vi "PPSU Feedback.vi"(8 "Error in":errorcluster, 11 "All Queue":T1) -> ()   [LabVIEW 2022 SP3]
uses:
  Controls/All Queue Ref.ctl
  Controls/PPSU Feedback ctl.ctl
  Controls/ALL Health.ctl
  6D_Global.vi
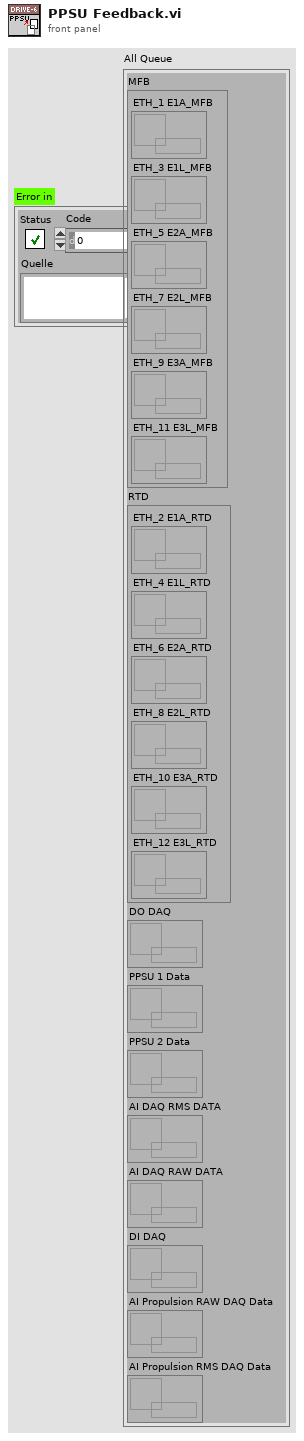
[diagram p1: front panel]
types:
  T1 = typedef "All Queue Ref.ctl" = cluster{"MFB":cluster{"ETH_1 E1A_MFB":refnum<queue>, "ETH_3 E1L_MFB":refnum<queue>, "ETH_5 E2A_MFB":refnum<queue>, "ETH_7 E2L_MFB":refnum<queue>, "ETH_9 E3A_MFB":refnum<queue>, "ETH_11 E3L_MFB":refnum<queue>}, "RTD":cluster{"ETH_2 E1A_RTD ":refnum<queue>, "ETH_4 E1L_RTD ":refnum<queue>, "ETH_6 E2A_RTD ":refnum<queue>, "ETH_8 E2L_RTD ":refnum<queue>, "ETH_10 E3A_RTD ":refnum<queue>, "ETH_12 E3L_RTD ":refnum<queue>}, "DO DAQ":refnum<queue>, "PPSU 1 Data":refnum<queue>, "PPSU 2 Data":refnum<queue>, "AI DAQ RMS DATA":refnum<queue>, "AI DAQ RAW DATA":refnum<queue>, "DI DAQ":refnum<queue>, "AI Propulsion RAW DAQ Data":refnum<queue>, "AI Propulsion RMS DAQ Data":refnum<queue>}
  T2 = typedef "PPSU Feedback ctl.ctl" = enum16{"Initialize", "Poll", "Read", "Exit"}
  T3 = typedef "ALL Health.ctl" = enum16{"AI HS", "AI 20kHZ HS", "DO HS", "Datalog HS", "PPSU HS", "ETH_1 DAQ", "ETH_1 RTD", "ETH_2 DAQ", "ETH_2 RTD", "ETH_5 RTD"}
  T4 = enum16{"Init", "Read 'All'", "Read 'n'", "Read '1'", "Write '1'", "Write 'n'", "Write 'All'"}
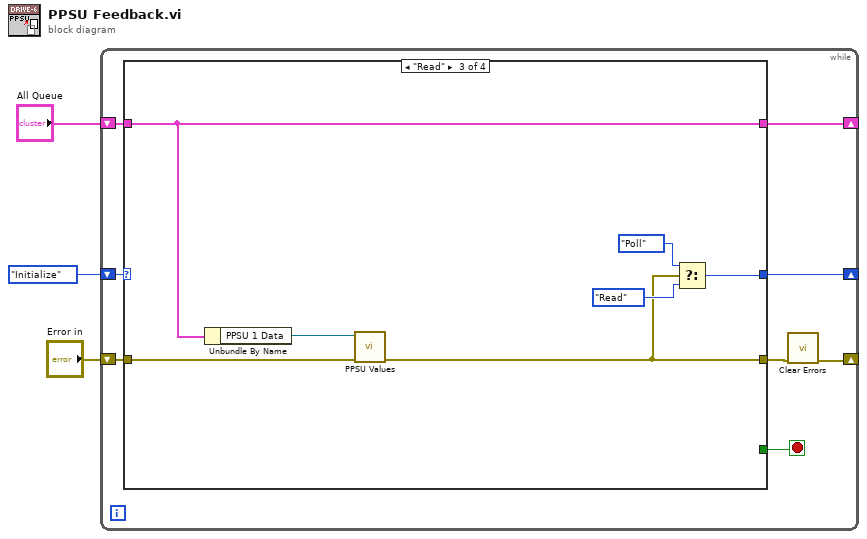
[diagram p0: block diagram]
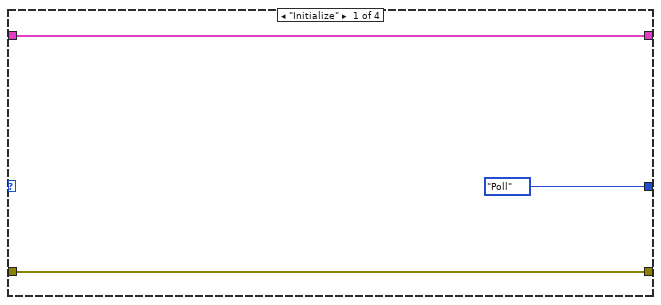
[diagram p2: hidden frame]
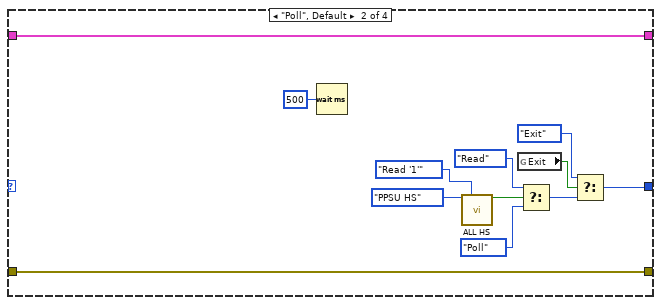
[diagram p3: hidden frame]
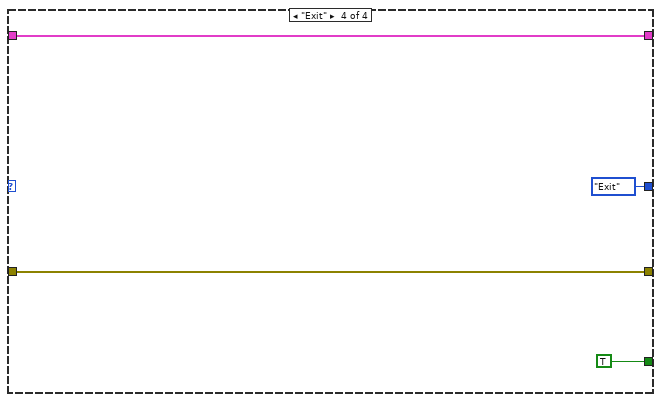
[diagram p4: hidden frame]
diagram:
  n1 = while {
    shift-right: [w10] -> _
    shift-left: PPSU_Feedback_ctl."Initialize" -> [w11]
    shift-right: [w7] -> _
    shift-left: "Error in" -> [w9]
    shift-right: [w4] -> _
    shift-left: "All Queue" -> [w5]
    stop <- w6 stop-if-true
    n2 = case shown="\"Read\"" w11 {
      tunnel: [PPSU_Feedback_ctl."Poll" w18 w30 PPSU_Feedback_ctl."Exit"] -> w10
      tunnel: w9 -> [w13 w16 w33 w37]
      tunnel: [w13 w16 w29 w37] -> w8
      tunnel: [_ _ _ TRUE] -> w6
      tunnel: w5 -> [w12 w15 w28 w34]
      tunnel: [w12 w15 w28 w34] -> w4
      frame "Initialize" {
      }
      frame "Poll", Default {
        n3 = Wait (ms)(milliseconds to wait=u32 500) -> ()  [unwired: 1 out]
        n4 = call "ALL HS.vi"("Loop"=ALL_Health."PPSU HS", "Option"=T4."Read '1'") -> ("Status Out"=w20:bool)  [unwired: 11 in, 2 out]
        n5 = global read "6D_Global.vi" "Exit"() -> (w24:bool)
        n6 = Select(t=PPSU_Feedback_ctl."Read", s=w20, f=PPSU_Feedback_ctl."Poll") -> (s? t:f=w19:T2)
        n7 = Select(t=PPSU_Feedback_ctl."Exit", s=w24, f=w19) -> (s? t:f=w18:T2)
      }
      frame "Read" {
        n8 = Unbundle By Name(w28) -> ("PPSU 1 Data"=w27:refnum<queue>)
        n9 = call "PPSU Values.vi"("error in"=w33, "PPSU Queue"=w27) -> ("Fehler"=w29:errorcluster)  [unwired: 9 in]
        n10 = Select(t=PPSU_Feedback_ctl."Poll", s=w29, f=PPSU_Feedback_ctl."Read") -> (s? t:f=w30:T2)
      }
      frame "Exit" {
      }
    }
    n11 = call <vilib>:"Clear Errors.vi"("error in (no error)"=w8) -> ("error out"=w7:errorcluster)  [unwired: 5 in, 1 out]
  }
